vi "SetParametrName.vi"(8 "error in (no error)":errorcluster, 9 "Значение":dbl, 10 "Имя параметра":i32(ring) items=["cp1", "cp2", "cp3", "cp4", "cp5", "cp6", "cp7", "cp8", "cp9", "cp10", "cp11", "cp12", "vp1", "vp2", "vp16", "vp3", "vp4", "vp5", "vp6", "vp7", "vp8", "vp9", "vp10", "vp11", "vp12", "vp13", "vp14", "vp15", "vp17", "vp18", "vp19", "vp20", "vp21", "vp22", "vp23", "vp24", "vp25", "vp26", "pp1", "pp2", "pp3", "pp5", "pp6", "pp7", "pp8", "pp9", "pp10", "pp11", "ss1", "ss2", "ss3", "ss4", "ss5", "ss6", "ss7", "ss8", "ss9", "ss10", "ss11", "ss12", "ss13", "ss14", "ss15", "si1", "si2", "ss16", "ss17", "ss18", "ct1", "ct2", "ct3", "dd1", "dd6", "dd3", "dd9", "dd2", "dd4", "dd5", "dd21", "dd7", "dd8", "dd20", "dd10", "dd19", "dd12", "dd11", "dd13", "dd14", "dd15", "dd16", "dd17", "dd18", "dd22", "dd23", "dd24", "dd25", "dd26", "dd27", "dd28", "dd29", "dd30", "dd31", "dd32", "dd33", "dd34", "st1", "st2", "st3", "st4", "st5", "st6", "st7", "st8", "st9", "st10", "st11", "st12", "st13", "st14", "tp1", "tp3", "tp2", "tp5", "tp6", "ip0", "ip1", "ip2", "ip3", "ip4", "ip5", "ip6", "ip7", "ip8", "ip9", "ip10", "ip11", "ip12", "ip13", "ip14", "ip15", "ip16", "ip17", "ip18", "ip19", "ip20", "ep1", "ep2", "ep3", "ep4", "ep5", "ep6", "ep7", "up0", "up1", "up2", "up3", "up4", "up5", "up6", "up7", "up8", "up9", "up10", "up11", "up12", "up13", "up14", "up15", "up16", "up17", "up18", "up19", "up20", "up21", "up22", "up23", "up24", "io0", "io1", "io2", "io3", "io4", "io5", "io6", "io7", "io8", "io9", "io10", "io11", "io12", "io13", "io14", "pd1", "pd2", "pd3", "pd4", "pd5", "pd6", "pd7", "pd8", "pd9", "pd10", "pd11", "pd12", "pd13", "pd14", "pd15", "pd16", "pd17", "pd18", "pd19"], 11 "StepMotor in":refnum<class "StepMotor.lvclass">) -> (0 "error out":errorcluster, 3 "StepMotor out":refnum<class "StepMotor.lvclass">)   [LabVIEW 2010, in "StepMotor.lvclass"]
uses:
  StepMotor.lvclass
  StepMotor.lvclass/StepMotor.ctl
panel:
  in  "Адреса параметров":u16(ring) items=["0000", "0002", "0004", "0005", "0010", "0048", "0053", "0060", "0814", "0815", "0821", "0822", "0006", "0007", "0050", "0008", "0009", "000A", "000E", "0011", "0014", "000F", "0031", "0032", "0033", "0034", "0039", "0040", "0063", "0A16", "0A17", "0A18", "0A19", "0A1A", "0A1B", "0A1C", "081F", "0820", "000B", "000C", "000D", "0012", "0041", "0A12", "0A13", "0A14", "0A15", "081C", "0013", "001F", "0020", "0021", "0022", "0023", "0024", "0025", "0026", "0027", "0028", "0029", "002A", "002B", "002C", "0600", "0601", "0818", "0819", "081A", "0200", "0202", "0204", "0400", "040A", "0405", "040D", "0402", "0408", "0409", "0419", "040B", "040C", "0418", "040E", "0417", "0410", "040F", "0411", "0412", "0413", "0414", "0415", "0416", "0420", "0421", "0422", "0423", "0424", "0425", "0426", "0427", "0428", "0429", "042A", "042B", "042C", "0015", "0016", "001E", "0046", "0047", "0802", "0804", "0062", "0816", "0817", "0823", "0824", "0825", "0826", "0500", "0504", "0502", "0505", "0506", "0017", "0018", "001A", "001B", "001C", "001D", "0030", "0035", "0036", "0037", "0038", "0042", "0045", "0057", "0058", "0059", "0061", "0800", "0801", "081D", "081E", "0043", "0044", "0051", "0052", "0054", "0056", "081B", "0700", "0701", "0702", "0703", "0704", "0705", "0706", "0707", "0708", "0709", "070A", "070B", "070C", "070D", "070E", "070F", "0710", "0711", "0712", "0713", "0714", "0715", "0716", "0717", "0718", "0805", "0806", "0807", "0808", "0809", "080A", "080B", "080C", "080D", "080E", "080F", "0810", "0811", "0812", "070F", "0A01", "0A02", "0A03", "0A04", "0A05", "0A06", "0A07", "0A08", "0A09", "0A0A", "0A0B", "0A0C", "0A0D", "0A0E", "0A0F", "0A10", "0A11", "0A1D", "0A1E", ""]
  in  "Чтение запись":u16(ring) items=["0", "0", "0", "0", "0", "0", "0", "0", "0", "0", "0", "0", "0", "0", "0", "0", "0", "0", "0", "0", "0", "0", "0", "0", "0", "0", "0", "0", "0", "0", "0", "0", "0", "0", "0", "0", "0", "0", "0", "0", "0", "0", "0", "0", "0", "0", "0", "0", "0", "0", "0", "0", "0", "0", "0", "0", "0", "0", "0", "0", "0", "0", "0", "0", "0", "0", "0", "0", "0", "0", "0", "1", "0", "1", "0", "1", "1", "1", "1", "1", "1", "1", "1", "1", "1", "0", "1", "1", "1", "1", "1", "1", "0", "1", "1", "1", "1", "1", "0", "1", "1", "1", "1", "1", "1", "0", "0", "0", "0", "0", "0", "0", "0", "0", "0", "0", "0", "0", "1", "0", "0", "0", "0", "0", "0", "0", "0", "1", "0", "0", "0", "0", "0", "0", "1", "1", "0", "0", "0", "0", "0", "0", "0", "0", "0", "0", "0", "0", "0", "0", "0", "0", "0", "0", "0", "0", "0", "0", "0", "0", "0", "0", "0", "0", "0", "0", "0", "0", "1", "0", "0", "0", "0", "0", "0", "0", "0", "0", "0", "0", "0", "0", "0", "0", "0", "0", "0", "0", "0", "0", "0", "1", "0", "0", "0", "0", "0", "0", "0", "0", "0", "0", "0", "0", "0", "0", "0", "1", "1", "0", "0", ""]
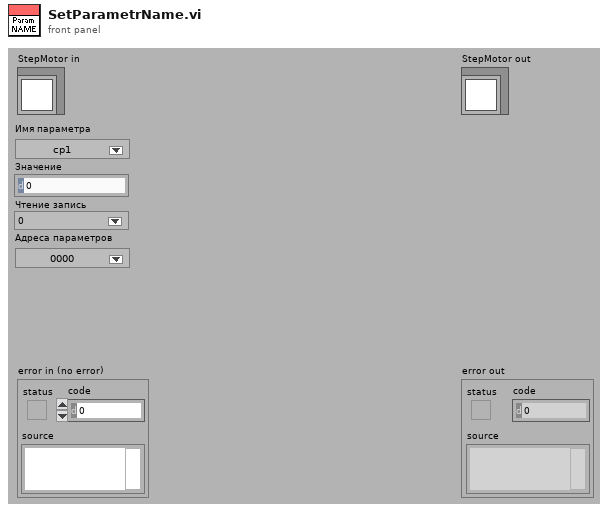
[diagram p1: front panel]
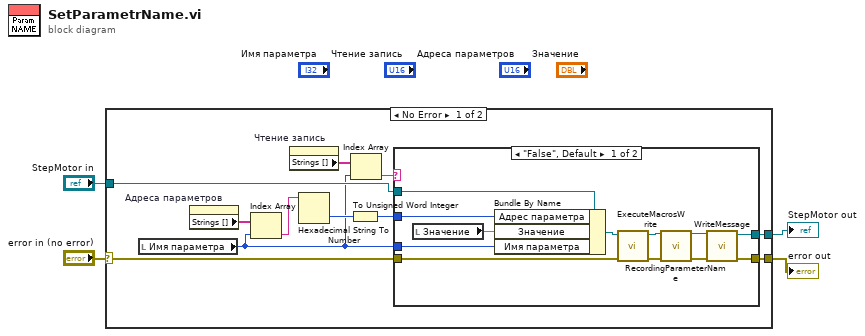
[diagram p0: block diagram]
diagram:
  n1 = case shown="No Error" "error in (no error)" {
    selector: "error in (no error)" -> [w13 w31]
    tunnel: [w14 w31] -> w3
    tunnel: [w15 w30] -> w1
    tunnel: "StepMotor in" -> [w12 w30]
    frame No Error {
      n2 = local read "Имя параметра"() -> (w6:i32)
      n3 = property on="Адреса параметров" class="Ring (strict)"() -> ("Strings []"=w11:string[])  [unwired: 2 in, 2 out]
      n4 = Index Array(array=w11, index=w6) -> (element=w10:string)
      n5 = property on="Чтение запись" class="Ring (strict)"() -> ("Strings []"=w7:string[])  [unwired: 2 in, 2 out]
      n6 = Hexadecimal String To Number(string=w10) -> (number=w9:u32)  [unwired: 2 in, 1 out]
      n7 = To Unsigned Word Integer(number=w9) -> (unsigned 16bit integer=w8:u16)
      n8 = Index Array(array=w7, index=w6) -> (element=w5:string)
      n9 = case shown="\"False\", Default" w5 {
        tunnel: [w17 w29] -> w15
        tunnel: [w16 w28] -> w14
        tunnel: w13 -> [w25 w28]
        tunnel: w8 -> [w24 _]
        tunnel: w6 -> [w23 _]
        tunnel: w12 -> [w21 w29]
        frame "False", Default {
          n10 = local read "Значение"() -> (w22:dbl)
          n11 = Bundle By Name(cluster=w21, "Адрес параметра"=w24, "Значение"=w22, "Имя параметра"=w23) -> (w20:refnum<class "StepMotor.lvclass">)
          n12 = call-dynamic "ExecuteMacrosWrite.vi"("error in (no error)"=w25, "StepMotor in"=w20) -> ("error out"=w26:errorcluster, "StepMotor out"=w27:refnum<class "StepMotor.lvclass">)  [unwired: 8 in]
          n13 = call "RecordingParameterName.vi"("StepMotor in"=w27, "error in (no error)"=w26) -> ("StepMotor out"=w19:refnum<class "StepMotor.lvclass">, "error out"=w18:errorcluster)  [unwired: 12 in]
          n14 = call-dynamic "WriteMessage.vi"("error in (no error)"=w18, "StepMotor in"=w19) -> ("error out"=w16:errorcluster, "StepMotor out"=w17:refnum<class "StepMotor.lvclass">)  [unwired: 8 in]
        }
        frame "True" {
        }
      }
    }
    frame Error {
    }
  }
  "error out" <- w3
  "StepMotor out" <- w1
